vi "calibration_for UI.vi"(8 "error in (no error)":errorcluster caption="错误输入（无错误）", 9 "parameter for calibration":T2={"分子长度（bp）"=0, "磁球大小（直径）"=0.0, "校准起点"=0.0, "校准步长"=0.0, "每步采样数（frame）"=0, "首尾去除帧数(frame)"=0, "校准步数"=0, "底面位置"=0.0, "R-step"=1.0, "R-min"=0.0, "R-max"=0.0, "num"=2, "x_center"=0.0, "y_center"=0.0, "磁铁位置"=0.0}, 10 "图像信号输入":dbl[][](array[numeric])) -> (0 "error out":errorcluster caption="错误输出", 2 "LUT":dbl[][][](array[numeric]))   [LabVIEW 2013]
doc: "使用该模板构建标准状态机设计模式。各状态执行代码并决定转移状态。将该设计模式与根据用户动作响应而执行代码的用户界面事件处理器模式相比较。同时将该设计模式与每段消息处理代码可以将零至多个新消息加入队列的队列消息处理器模式相比较。\n注：该模板的设计未遵守最新NI推荐的编程风格。请通过“创建项目”对话框（而不要采用该模板），创建基于项目的标准状态机模式的完整实现。"
uses:
  cali_state.ctl
  parameter set for calibration.ctl
  parameter for radial profile.ctl
panel:
  in  "parameter for radial profile":T1={"R-step"=1.0, "R-min"=0.0, "R-max"=0.0, "num"=2, "x_center"=0.0, "y_center"=0.0, "校准起点"=0.0, "校准步长"=0.0, "校准终点"=0.0, "每步采样数（frame）"=0, "首尾去除帧数(frame)"=0, "Array R"=[], "Array profile"=[]}
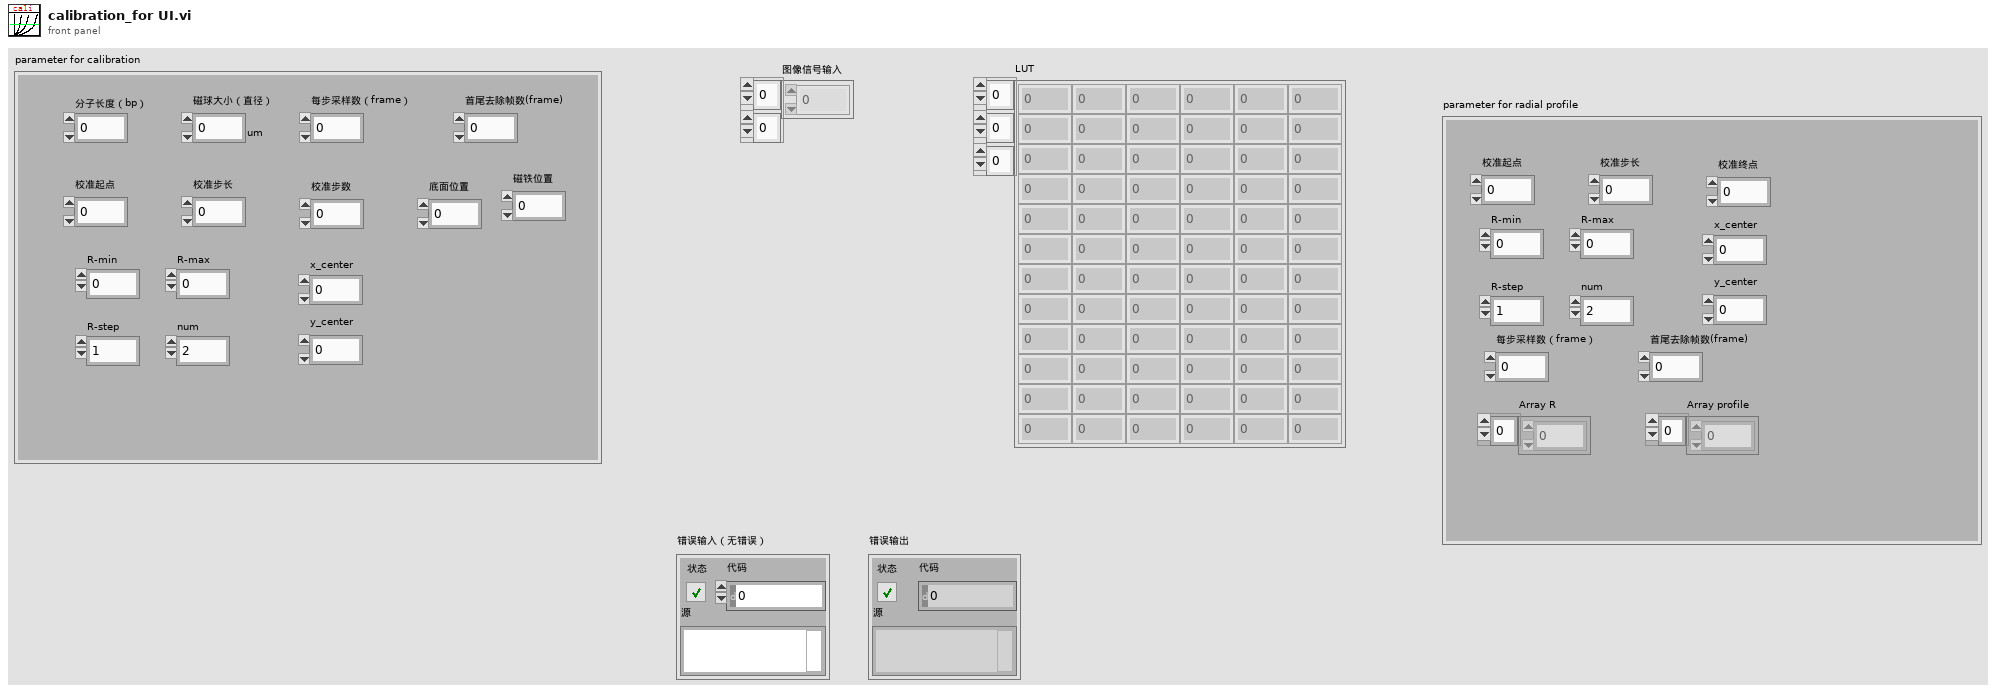
[diagram p1: front panel]
types:
  T1 = typedef "parameter for radial profile.ctl" = cluster{"R-step":sgl, "R-min":sgl, "R-max":sgl, "num":i32, "x_center":dbl, "y_center":dbl, "校准起点":dbl, "校准步长":dbl, "校准终点":dbl, "每步采样数（frame）":i32, "首尾去除帧数(frame)":i32, "Array R":dbl[], "Array profile":dbl[]}
  T2 = typedef "parameter set for calibration.ctl" = cluster{"分子长度（bp）":i32, "磁球大小（直径）":dbl[unit], "校准起点":dbl, "校准步长":dbl, "每步采样数（frame）":i32, "首尾去除帧数(frame)":i32, "校准步数":i32, "底面位置":dbl, "R-step":sgl, "R-min":sgl, "R-max":sgl, "num":i32, "x_center":dbl, "y_center":dbl, "磁铁位置":dbl}
  T3 = typedef "cali_state.ctl" = enum16{"Initialize", "LUT determined", "generate LUT"}
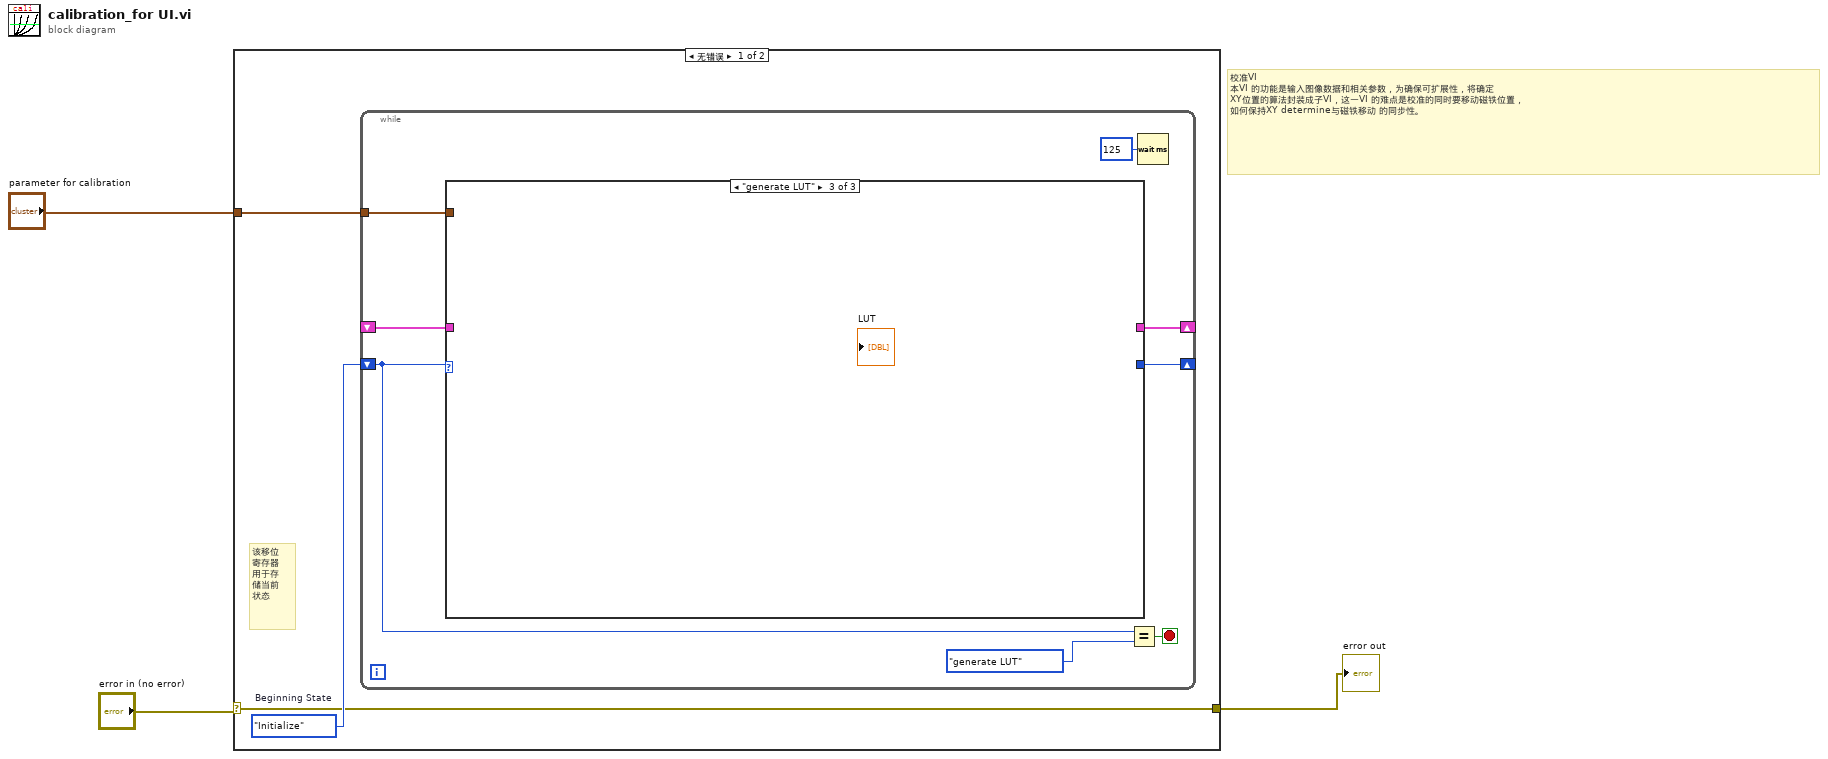
[diagram p0: block diagram]
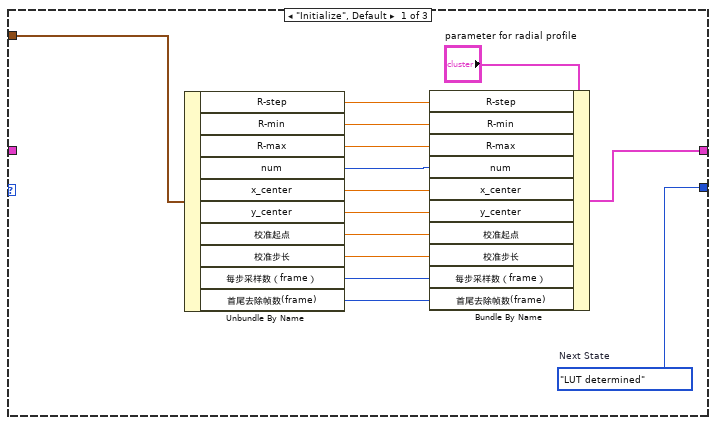
[diagram p2: hidden frame]
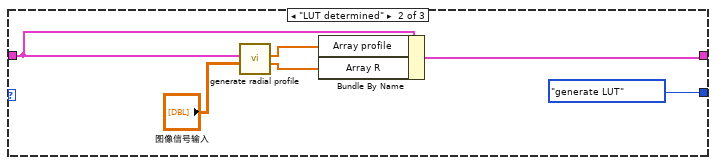
[diagram p3: hidden frame]
diagram:
  # "校准VI\n本VI 的功能是输入图像数据和相关参数，为确保可扩展性，将确定\nXY位置的算法封装成子VI，这一VI 的难点是校准的同时要移动磁铁位置，\n如何保持XY determine与磁铁移动 的同步性。"
  n1 = case shown="无错误" "error in (no error)" {
    selector: "error in (no error)" -> [w5 w35]
    tunnel: [w5 w35] -> w2
    tunnel: "parameter for calibration" -> [w4 _]
    frame No Error {
      w6 = cali_state."Initialize"  # Beginning State
      # "该移位\n寄存器\n用于存\n储当前\n状态"
      n2 = while {
        shift-right: [w11] -> _
        shift-left: w6 -> [w12]
        shift-right: [w8] -> _
        shift-left: _ -> [w9]
        tunnel: w4 -> [w7]
        stop <- w14 stop-if-true
        n3 = case shown="\"generate LUT\"" w12 {
          tunnel: [w28 cali_state."generate LUT" ("Next State") _] -> w11
          tunnel: w9 -> [_ w32 _]
          tunnel: [w26 w29 _] -> w8
          tunnel: w7 -> [w27 _ _]
          frame "Initialize", Default {
            w28 = cali_state."LUT determined"  # Next State
            n4 = Unbundle By Name(w27) -> ("R-step"=w24:sgl, "R-min"=w23:sgl, "R-max"=w22:sgl, "num"=w21:i32, "x_center"=w20:dbl, "y_center"=w19:dbl, "校准起点"=w18:dbl, "校准步长"=w17:dbl, "每步采样数（frame）"=w16:i32, "首尾去除帧数(frame)"=w15:i32)
            n5 = Bundle By Name(cluster="parameter for radial profile", "R-step"=w24, "R-min"=w23, "R-max"=w22, "num"=w21, "x_center"=w20, "y_center"=w19, "校准起点"=w18, "校准步长"=w17, "每步采样数（frame）"=w16, "首尾去除帧数(frame)"=w15) -> (w26:T1)
          }
          frame "LUT determined" {
            n6 = call "generate radial profile.vi"("图像信号"="图像信号输入", "parameter for radial profile"=w32) -> ("ArrayR"=w30:sgl[], "profile"=w31:dbl[])  [unwired: 7 in, 1 out]
            n7 = Bundle By Name(cluster=w32, "Array profile"=w31, "Array R"=w30) -> (w29:T1)
          }
          frame "generate LUT" {
          }
        }
        n8 = Equal?(x=w12, y=cali_state."generate LUT" ("States")) -> (x = y?=w14:bool)
        n9 = Wait (ms)(milliseconds to wait=u32 125) -> ()  [unwired: 1 out]
      }
    }
    frame Error {
    }
  }
  "error out" <- w2
